vi "MON.vi"(4 "error in (no error)":errorcluster, 7 "connection ID":refnum<k5>) -> (0 "error out":errorcluster, 3 "connection ID out":refnum<k5>)   [LabVIEW 2025, in "CAENels FAST-PS.lvlib"]
doc: "The MON (Module ON) command turns ON the FAST-PS output driver, thus enabling the output terminals and allowing the power supply to regulate and feed current or voltage to the connected load.\nAfter the reception of a \"MON\" command, the power supply automatically sets output current to 0A or 0V (depending if the module is set in constant current or constant voltage mode)."
uses:
  CAENels FAST-PS.lvlib
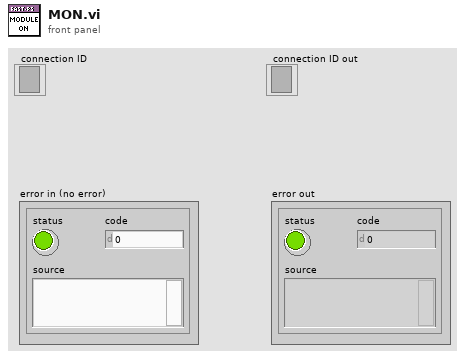
[diagram p1: front panel]
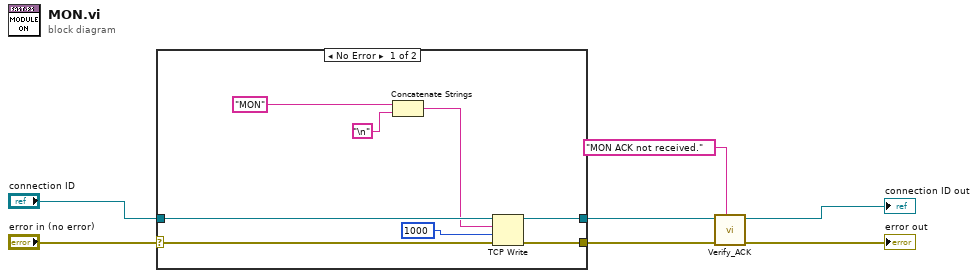
[diagram p0: block diagram]
diagram:
  n1 = case shown="No Error" "error in (no error)" {
    selector: "error in (no error)" -> [w15 w17]
    tunnel: [w14 w17] -> w5
    tunnel: [w13 w16] -> w3
    tunnel: "connection ID" -> [w12 w16]
    frame No Error {
      n2 = Concatenate Strings("MON" ("string (\"\")"), "\n") -> (w10:string)
      n3 = TCP Write(connection ID=w12, data in=w10, error in (no error)=w15, 9:1000 ("timeout ms (25000)")) -> (connection ID out=w13:refnum<k5>, error out=w14:errorcluster)  [unwired: 1 out]
    }
    frame Error {
    }
  }
  n4 = call "Verify_ACK.vi"("error code description"="MON ACK not received.", "error in (no error)"=w5, "connection ID"=w3) -> ("error out"=→"error out":errorcluster, "connection ID out"=→"connection ID out":refnum<k5>)  [unwired: 5 in]
